vi "Create.vi"(7 "mode settings":variant, 8 "error in":errorcluster, 9 "number of default channels":i32, 10 "channel settings":variant, 11 "pwm mode in":refnum<class "PWM Mode.lvclass">) -> (0 "error out":errorcluster, 1 "channels":refnum<class "Channel.lvclass">[](array[class]), 3 "pwm mode out":refnum<class "PWM Mode.lvclass">)   [LabVIEW 2017, in "Scan Engine Scripting.lvlib" / "PWM Mode.lvclass"]
uses:
  PWM Mode.lvclass
  Channel Classes/Channel/Channel.lvclass
  Controls/pwm channel settings.ctl
  Channel Classes/PWM Output Channel/Frequency.ctl
  e5b725c6-3e0b-4167-a346-9cfd727ed9ab.vi
  Channel Classes/PWM Output Channel/PWM Output Channel.lvclass
  C:/dev/github.com/debryant/niveristand-scan-engine-ethercat-custom-device/Custom Device Source/Scripting/Modules/Channel Classes/Channel/Channel.lvclass
  Scan Engine Scripting.lvlib
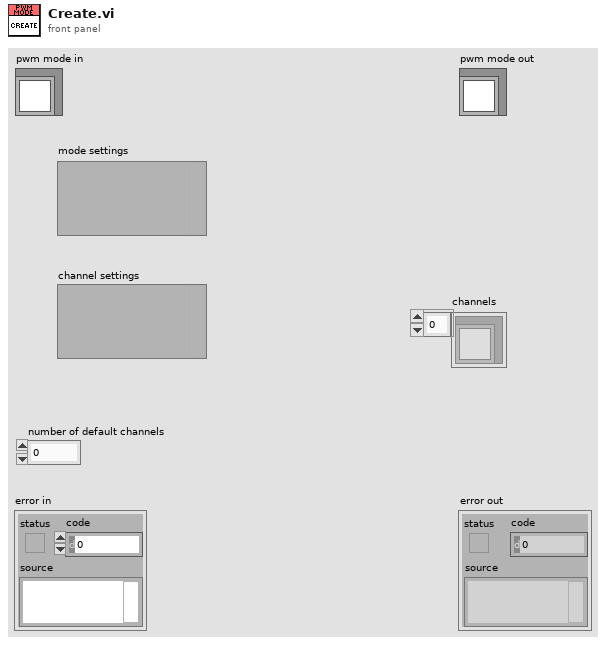
[diagram p1: front panel]
types:
  T1 = typedef "Scan Engine Scripting.lvlib/pwm channel settings.ctl" = cluster{"name":string, "default value":dbl, "frequency":T2}
  T2 = typedef "Scan Engine Scripting.lvlib/PWM Output Channel.lvclass/Frequency.ctl" = enum16{"1 Hz (1,000,000 us)", "50 Hz (20,000 us)", "250 Hz (4,000 us)", "500 Hz (2,000 us)", "1 kHz (1,000 us)", "5 kHz (200 us)", "10 kHz (100 us)", "20 kHz (50 us)"}
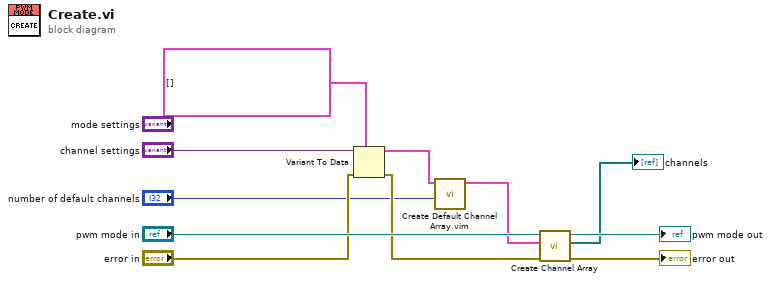
[diagram p0: block diagram]
diagram:
  n1 = Variant To Data(error in="error in", type=T1[] [] ("channel settings"), Variant="channel settings") -> (data=w2:T1[], error out=w5:errorcluster)
  n2 = call "Create Default Channel Array.vim"("number of default channels"="number of default channels", "channel settings in"=w2) -> ("channel settings out"=w1:T1[])  [unwired: 9 in]
  n3 = call "Create Channel Array.vi"("error in"=w5, "channel settings"=w1, "PWM Mode in"="pwm mode in") -> ("error out"=→"error out":errorcluster, "channels"=→"channels":refnum<class "PWM Output Channel.lvclass">[], "PWM Mode out"=→"pwm mode out":refnum<class "PWM Mode.lvclass">)  [unwired: 6 in]
